vi "Example_OE1311&OE1351 Trig in.vi"() -> ()   [LabVIEW 2011]
panel:
  in  "Parameter Index":u16(ring) items=["X", "Y", "R", "θ", "XD1", "YD1", "RD1", "θD1", "XD2", "YD2", "RD2", "θD2", "XD3", "YD3", "RD3", "θD3", "XD4", "YD4", "RD4", "θD4", "XD5", "YD5", "RD5", "θD5", "XD6", "YD6", "RD6", "θD6", "XD7", "YD7", "RD7", "θD7", "X_Noise", "Y_Noise", "Frequency", "AUX-IN1", "AUX-IN2"]
  in  "Trig Mode":u8(ring) items=["Ext_Rissing_Edge", "Ext_Falling_Edge", "Ext_Bilateral_Edge", "Ext_High_Level", "Ext_Low_Level"]
  in  "Trig Source":u8(ring) items=["Internal", "Aux-in1", "Aux-in2"]
  out "Wave":dbl(graph)
  out "loss count":i32=-1
  out "Group":u32
  out "Error out":errorcluster caption="error out"
  in  "function":T1(ring)
  in  "Connect":bool
  in  "Port":u32=10001
  in  "Timeout":u32=100
  in  "IP Address":string="192.168.1.1"
  in  "选项卡控件":enum32{"选项卡 "}(tab)
  in  "Sweep Mode":u16(ring) items=["Linear", "Log"]
  in  "Start Frequency(Hz)":dbl=1000.0 min=1e-05 max=60000000.0 format="%#.3f"
  in  "Stop Frequency(Hz)":dbl=5000.0 min=1e-05 max=60000000.0 format="%#.3f"
  in  "Linear Step Frequency(Hz)":dbl=1000.0 min=1e-05 max=60000000.0 format="%#.3f"
  in  "Log Step Percent(%)":dbl=10.0 min=-100.0 max=100.0 format="%#.2f"
  in  "Step Time(ms)":i32=1000 min=50 max=100000
  in  "Sweep Run Mode":u16(ring) items=["Stop", "Singal", "Loop"]
  in  "Interval Count":u32=1 min=1 max=100000
  in  "Ref_Source":u8(ring) items=["External", "Internal"]
  in  "Sweep":u16(ring) items=["OFF", "ON"]
  out "data_buffer":dbl[][](array[numeric])
  out "cnt":u16
  # "Tel          :   +86-020-84133345\nWebsite  :   www.ssi-instrument.com\nE-mail     :   support@si-instrument.com"
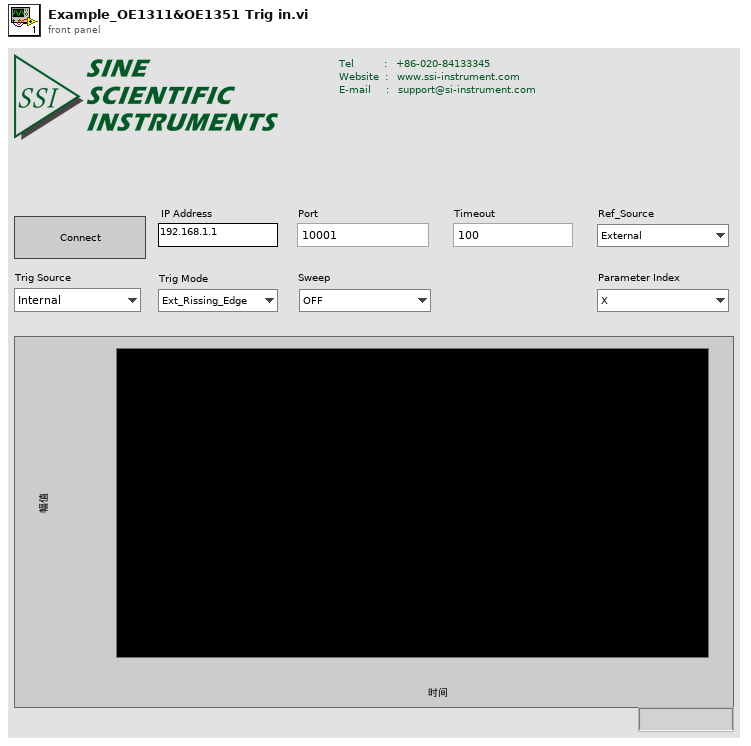
[diagram p1: front panel]
types:
  T1 = enum16{"initial", "Trig In Type", "Sample", "Ext_Sweep_Trig In", "Int_Sweep_Trig In"}
  T2 = enum8{"Enabled", "Disabled", "Disabled and Grayed Out"}
  T3 = cluster{"Port":u32, "Timeout":u32, "IP Address":string}
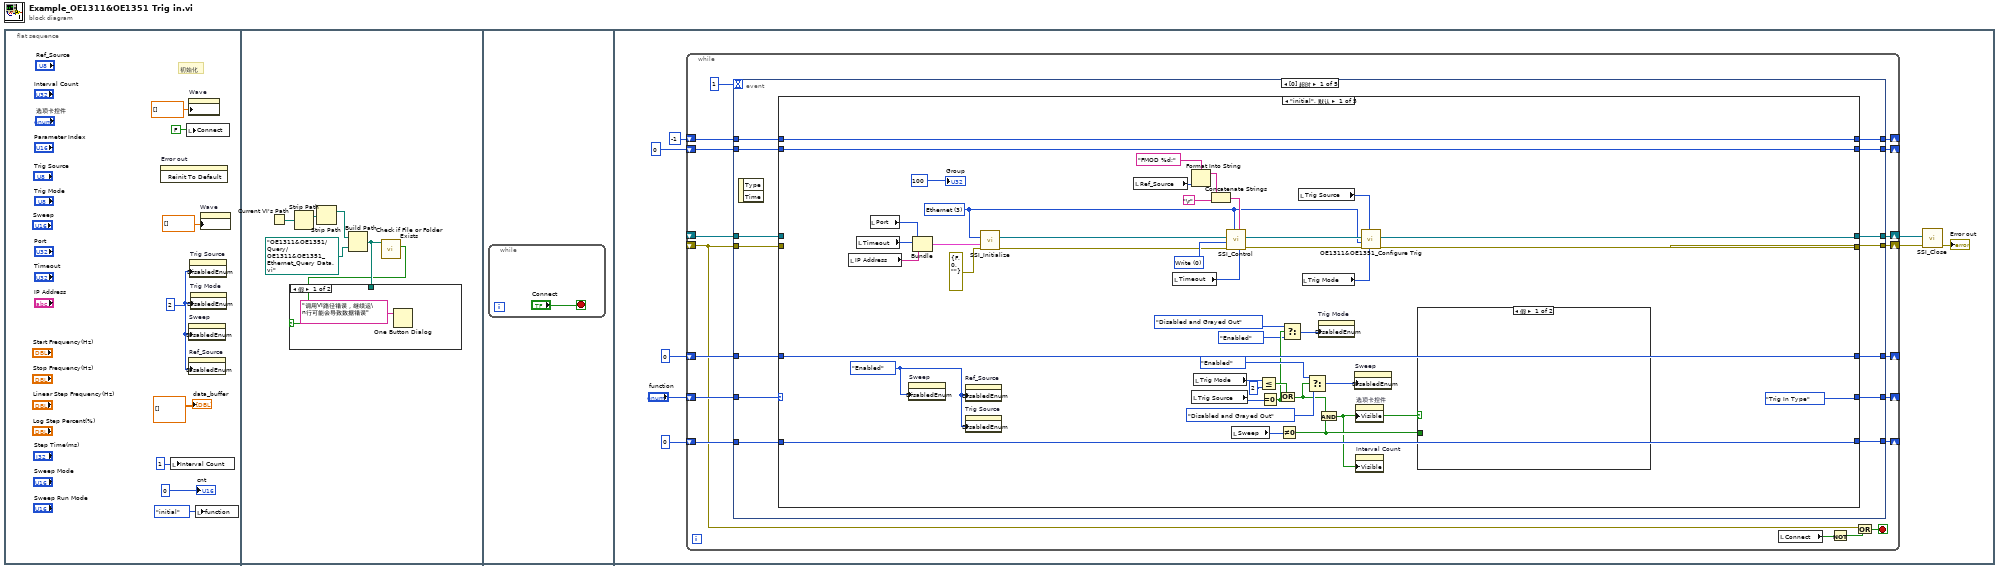
[diagram p0: block diagram]
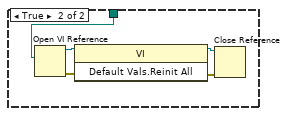
[diagram p2: hidden frame]
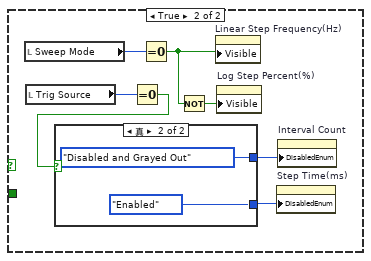
[diagram p3: hidden frame]
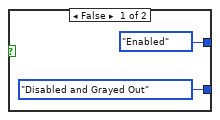
[diagram p4: hidden frame]
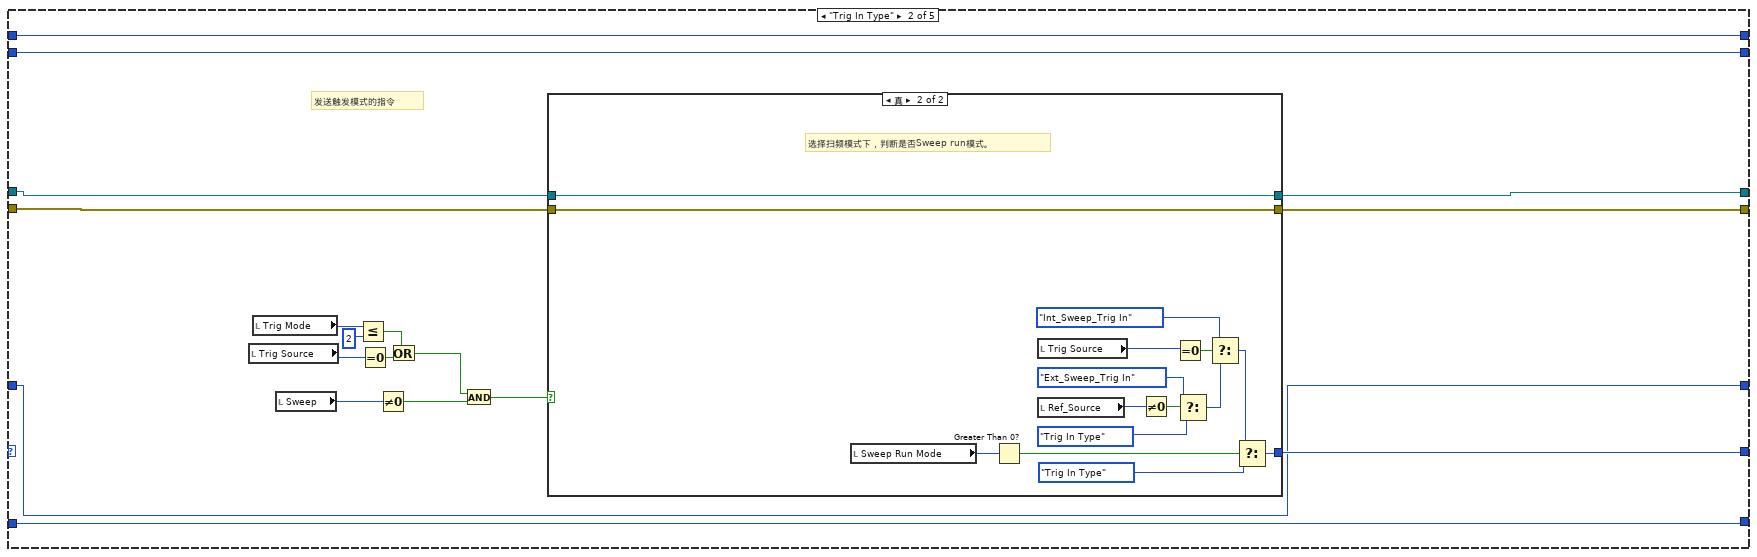
[diagram p5: hidden frame]
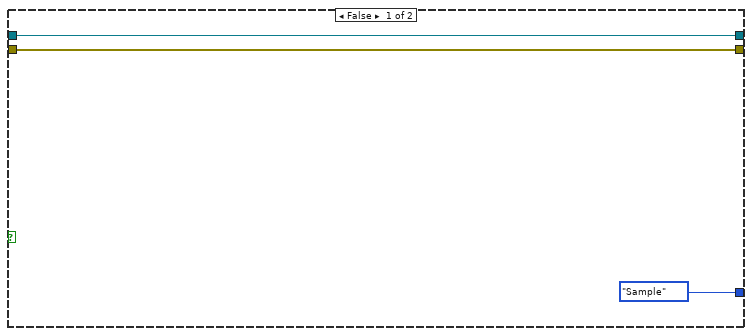
[diagram p6: hidden frame]
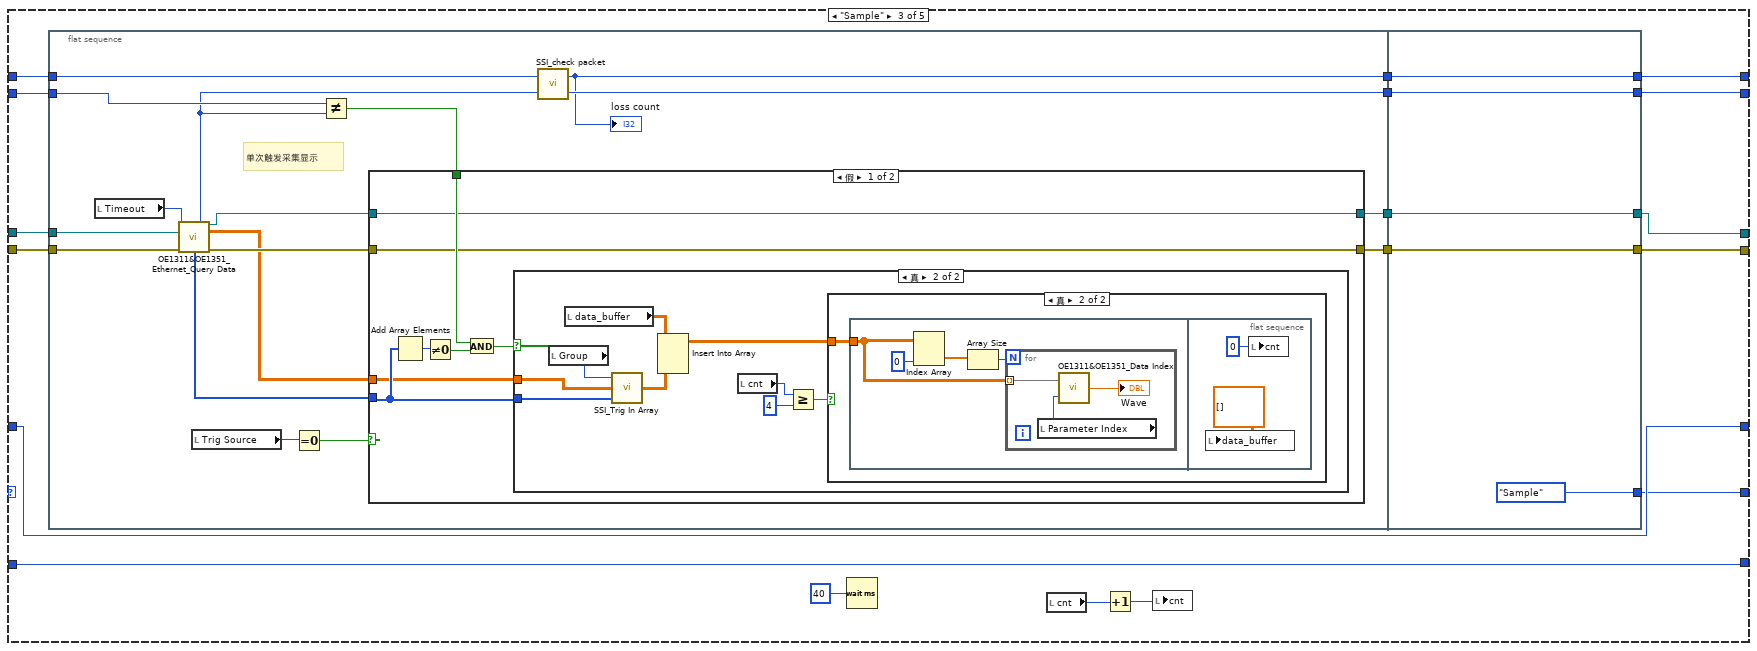
[diagram p7: hidden frame]
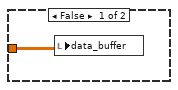
[diagram p9: hidden frame]
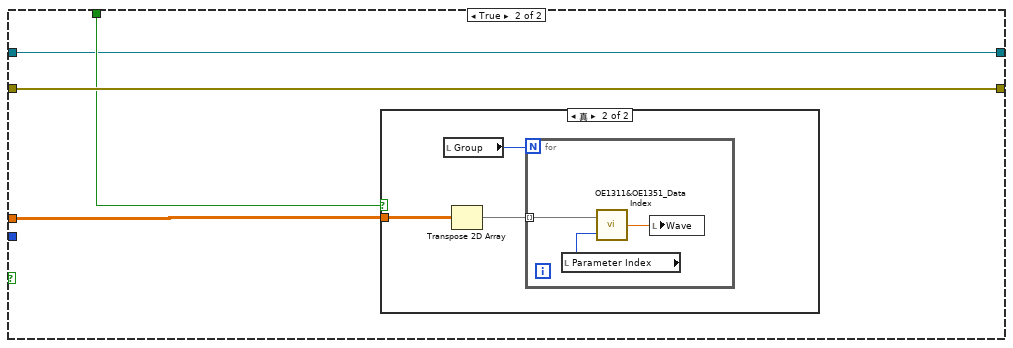
[diagram p10: hidden frame]
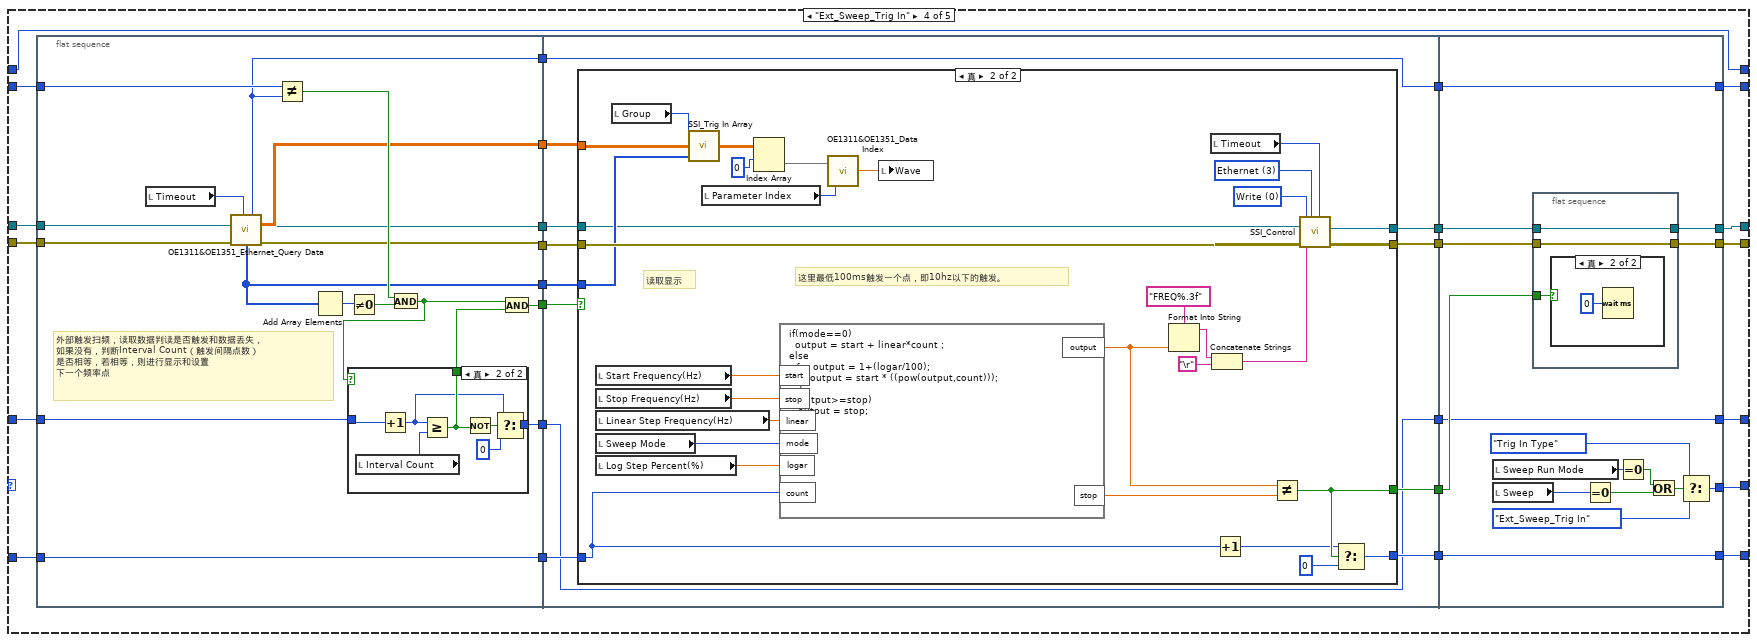
[diagram p12: hidden frame]
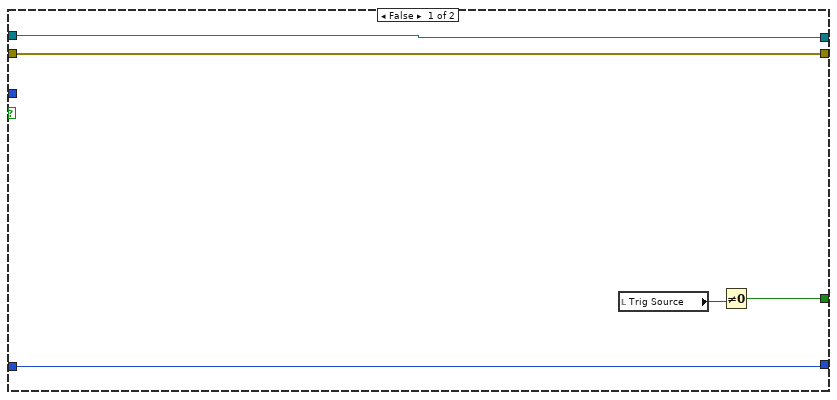
[diagram p14: hidden frame]
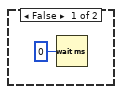
[diagram p15: hidden frame]
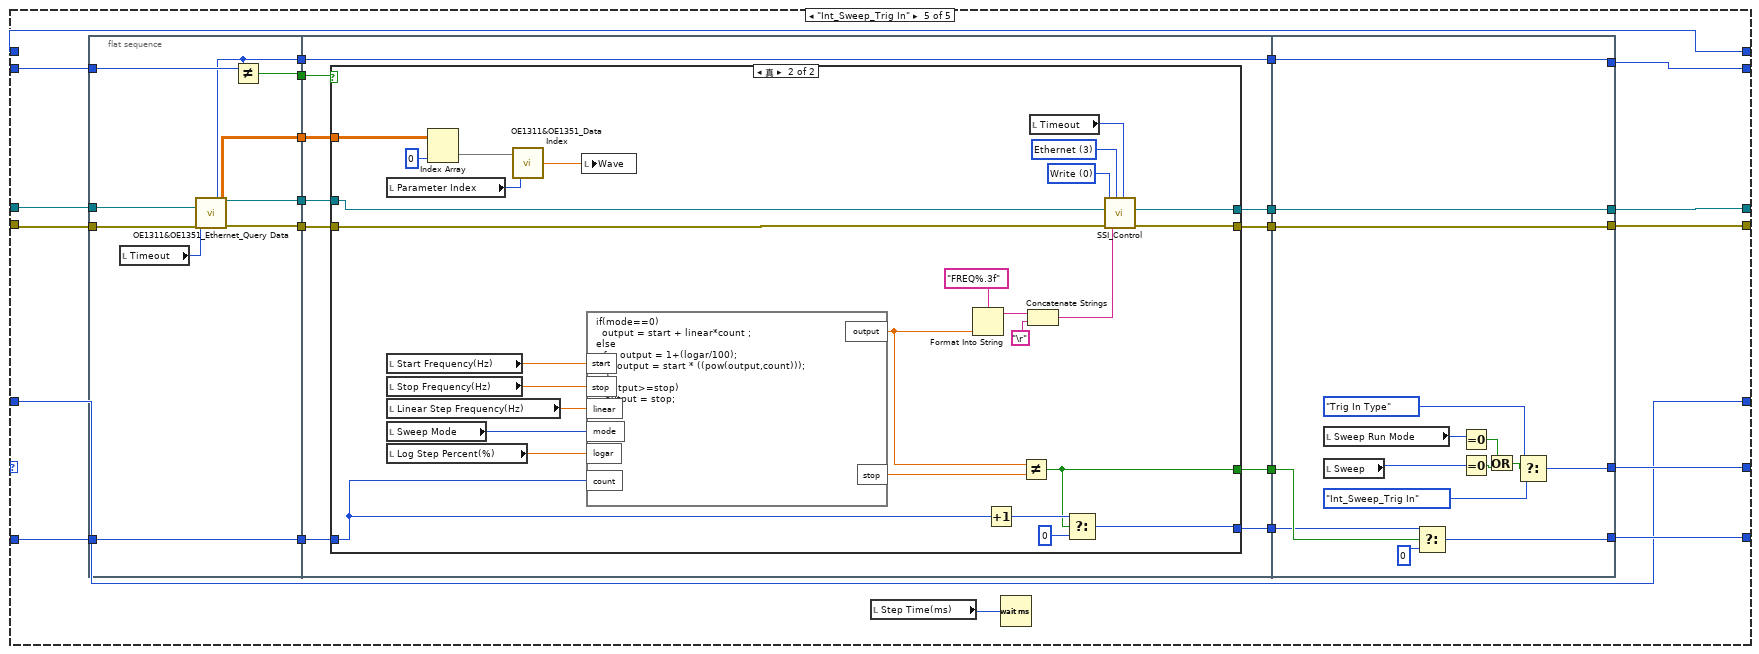
[diagram p16: hidden frame]
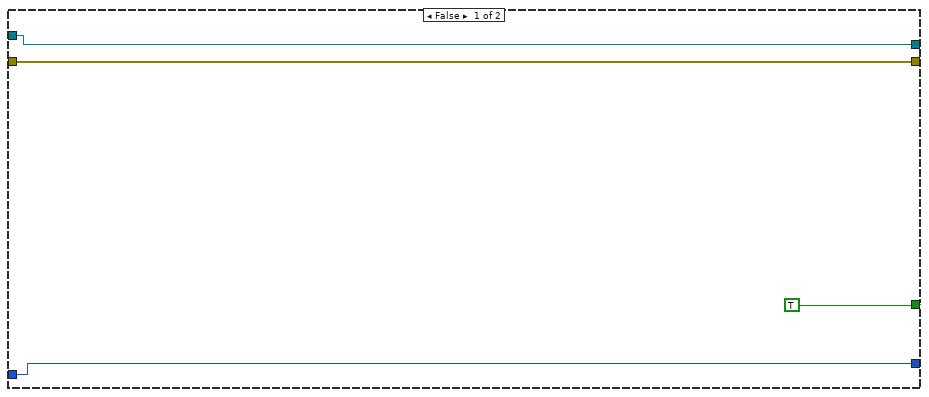
[diagram p17: hidden frame]
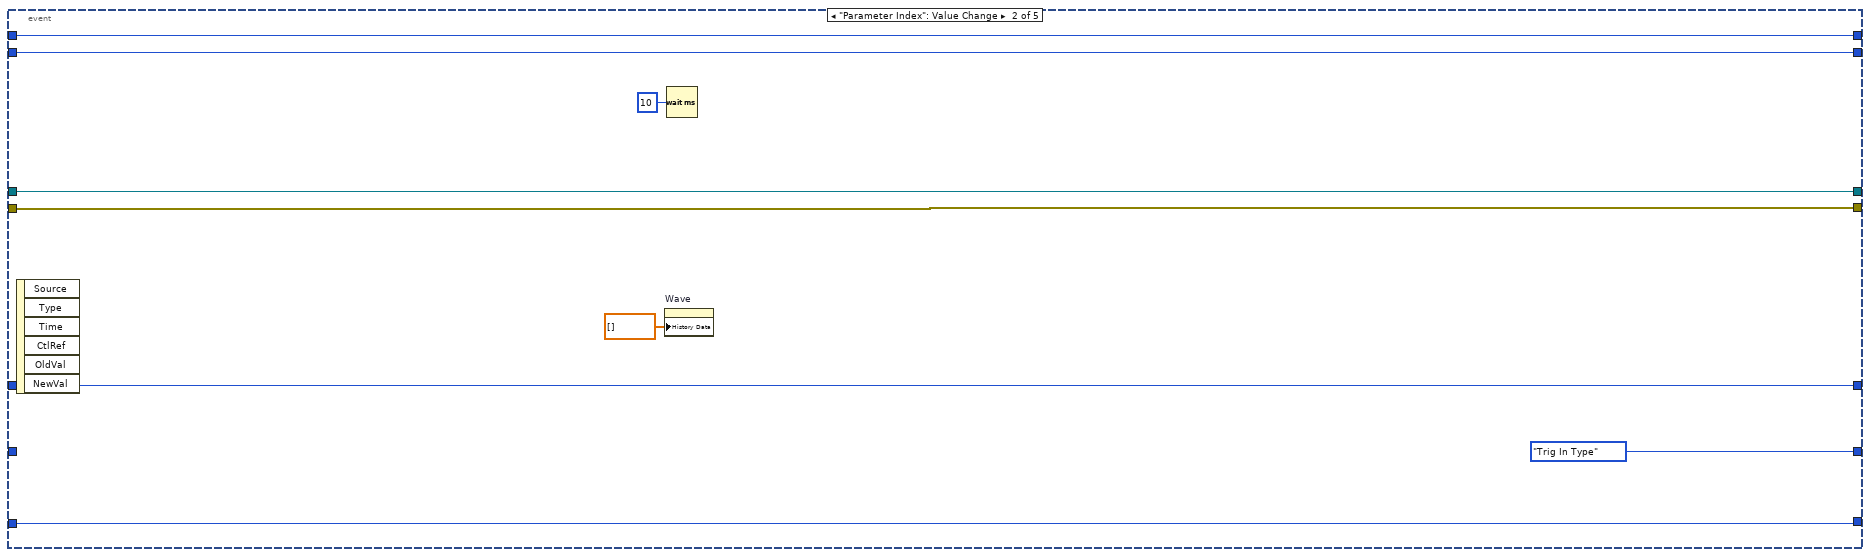
[diagram p18: hidden frame]
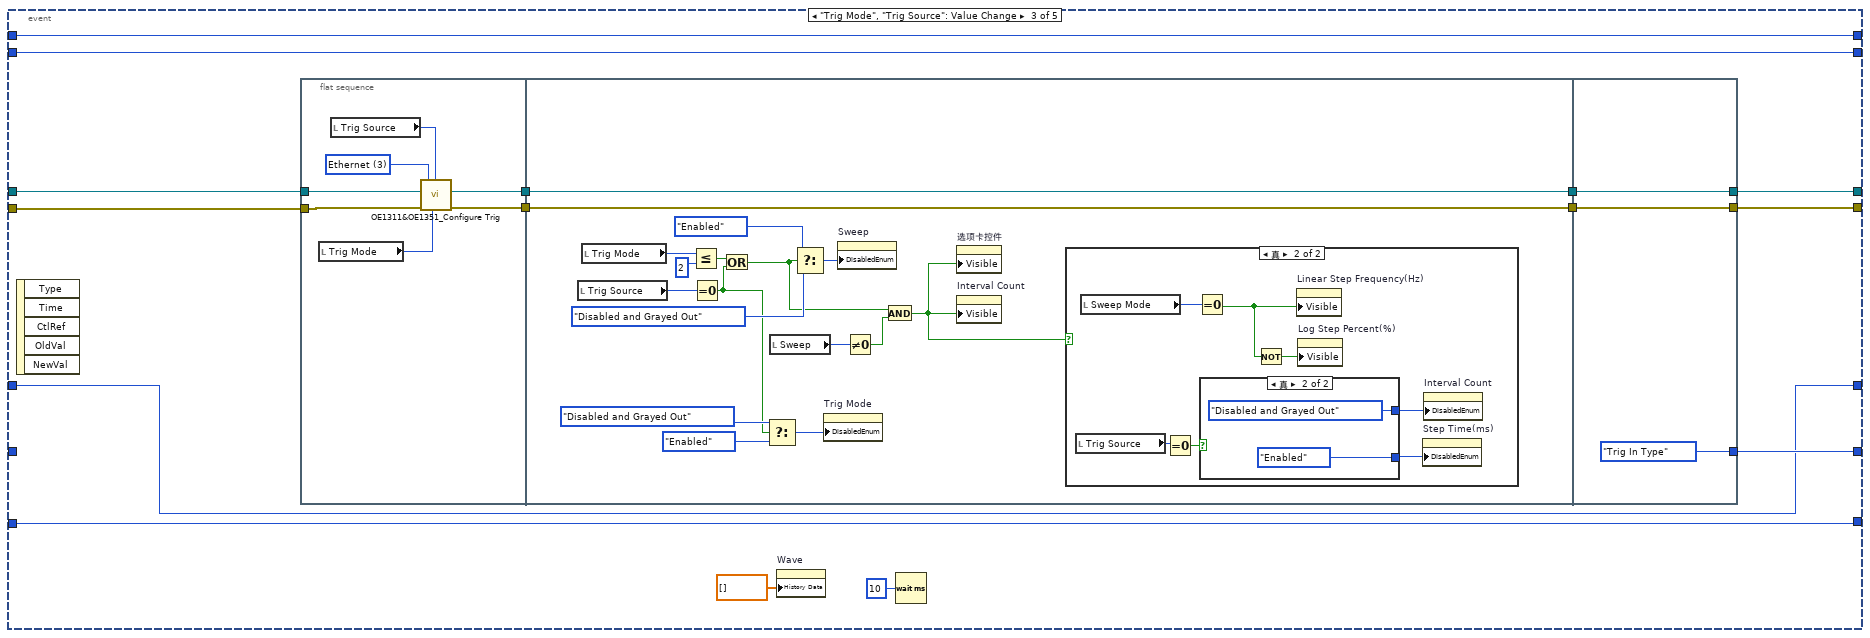
[diagram p19: hidden frame]
diagram:
  n1 = flat-sequence {
    frame #0 {
      w1 = 2
      # "初始化"
      n2 = invoke on="Error out" class="Clust (严格)" method="Reinit To Default"() -> ()  [unwired: 3 in, 3 out]
      n3 = local write "Interval Count"(u32 1 ("Interval Count")) -> ()
      n4 = local write "Connect"(FALSE ("Connect")) -> ()
      n5 = property on="Wave" class="WFChart (严格)"("History Data"=dbl[] [] ("历史数据")) -> ()  [unwired: 2 in, 2 out]
      n6 = property on="Sweep" class="Ring (严格)"("DisabledEnum"=w1) -> ()  [unwired: 2 in, 2 out]
      n7 = property on="Ref_Source" class="Ring (严格)"("DisabledEnum"=w1) -> ()  [unwired: 2 in, 2 out]
      n8 = property on="Trig Source" class="Ring (严格)"("DisabledEnum"=w1) -> ()  [unwired: 2 in, 2 out]
      n9 = property on="Trig Mode" class="Ring (严格)"("DisabledEnum"=w1) -> ()  [unwired: 2 in, 2 out]
      n10 = local write "function"(T1."initial" ("function")) -> ()
      n11 = property on="Wave" class="WFChart (严格)"("History Data"=dbl[] [] ("历史数据")) -> ()  [unwired: 2 in, 2 out]
      "data_buffer" <- dbl[][] []
      "cnt" <- 0
    }
    frame #1 {
      n12 = Current VI's Path() -> (path=w10:path)
      n13 = Strip Path(path=w10) -> (stripped path=w9:path)  [unwired: 1 out]
      n14 = Strip Path(path=w9) -> (stripped path=w11:path)  [unwired: 1 out]
      n15 = Build Path(base path=w11, name or relative path=path "OE1311&OE1351/Query/OE1311&OE1351_Ethernet_Query Data.vi") -> (appended path=w14:path)
      n16 = call <vilib>:"Check if File or Folder Exists.vi"("path"=w14) -> ("file or folder exists?"=w12:bool)  [unwired: 8 in, 2 out]
      n17 = case shown="假" w12 {
        tunnel: w14 -> [_ w20]
        frame False {
          n18 = One Button Dialog(message="调用VI路径错误，继续运\n行可能会导致数据错误" ("消息")) -> ()  [unwired: 1 in, 1 out]
        }
        frame True {
          n19 = Open VI Reference(vi path=w20) -> (vi reference=w17:refnum<vi>, error out=w16:errorcluster)  [unwired: 5 in]
          n20 = invoke class="VI" method="Default Vals.Reinit All"(reference=w17, error in=w16) -> (reference out=w19:refnum<vi>, error out=w18:errorcluster)  [unwired: 1 in, 1 out]
          n21 = Close Reference(reference=w19, error in (no error)=w18) -> ()  [unwired: 1 out]
        }
      }
    }
    frame #2 {
      n22 = while {
        stop <- "Connect" stop-if-true
      }
    }
    frame #3 {
      n23 = while {
        shift-right: [w43] -> _
        shift-left: "function" -> [w44]
        shift-right: [w41] -> _
        shift-left: 0 ("f") -> [w42]
        shift-right: [w38] -> _
        shift-left: 0 -> [w39]
        shift-right: [w35] -> _
        shift-left: 0 -> [w36]
        shift-right: [w45] -> w28
        shift-left: _ -> [w34]
        shift-right: [w33] -> w24
        shift-left: _ -> [w32]
        shift-right: [w30] -> _
        shift-left: -1 ("loss count") -> [w31]
        stop <- w46 stop-if-true
        n24 = event shown="[0] 超时" {
          selector: _ -> [_ _ _ _ _]
          dyn-events: _ -> [_ _ _ _ _]
          timeout: 1 -> [_ _ _ _ _]
          tunnel: [w61 w446 w452 w509 w526] -> w45
          tunnel: w34 -> [w60 w446 w456 w510 w526]
          tunnel: w44 -> [w59 _ _ w513 _]
          tunnel: [w58 T1."Trig In Type" ("function") w458 w513 T1."Trig In Type" ("function")] -> w43
          tunnel: w42 -> [w57 w448 w463 w514 w522]
          tunnel: [w56 w448 w463 w514 w522] -> w41
          tunnel: w39 -> [w55 w444 w462 w511 w524]
          tunnel: [w54 w444 w462 w511 w524] -> w38
          tunnel: w36 -> [w53 w443 w457 w512 w521]
          tunnel: [w52 w443 w457 w512 w521] -> w35
          tunnel: [w51 w441 w449 w507 w525] -> w33
          tunnel: w32 -> [w50 w441 w455 w508 w525]
          tunnel: w31 -> [w49 w440 w459 w503 w523]
          tunnel: [w48 w440 w459 w503 w523] -> w30
          event Timeout {
            n25 = event-data() -> ()  [unwired: 1 in, 2 out]
            n26 = case shown="\"initial\", 默认" w59 {
              tunnel: w60 -> [_ w133 w168 w254 w360]
              tunnel: [w93 w132 w161 w252 w370] -> w61
              tunnel: [T1."Trig In Type" ("function") w131 w166 w243 w368] -> w58
              tunnel: w57 -> [w103 w130 w169 w253 w369]
              tunnel: [w103 w130 w169 w251 w367] -> w56
              tunnel: w55 -> [w101 w129 w165 w250 w372]
              tunnel: [w101 w129 w163 w249 w371] -> w54
              tunnel: w53 -> [w102 w128 w167 w237 w366]
              tunnel: [w102 w128 w167 w234 w366] -> w52
              tunnel: [w94 w123 w154 w231 w352] -> w51
              tunnel: w50 -> [_ w124 w156 w233 w356]
              tunnel: w49 -> [w85 w122 w159 w230 w351]
              tunnel: [w85 w122 w153 w230 w351] -> w48
              frame "initial", Default {
                w64 = u16 3 items=["USB", "RS232", "GPIB", "Ethernet"] ("Remote Mode")
                w82 = T2."Enabled" ("禁用")
                w87 = u16 0 items=["Write", "Read"] ("Control")
                n27 = local read "IP Address"() -> (w90:string)
                n28 = local read "Timeout"() -> (w91:u32)
                n29 = local read "Port"() -> (w92:u32)
                n30 = property on="Sweep" class="Ring (严格)"("DisabledEnum"=w82) -> ()  [unwired: 2 in, 2 out]
                n31 = Bundle("Port"=w92, "Timeout"=w91, "IP Address"=w90) -> (w89:T3)  [unwired: 1 in]
                n32 = property on="Ref_Source" class="Ring (严格)"("DisabledEnum"=w82) -> ()  [unwired: 2 in, 2 out]
                n33 = property on="Trig Source" class="Ring (严格)"("DisabledEnum"=w82) -> ()  [unwired: 2 in, 2 out]
                n34 = call "SSI_Initialize.vi"("Remote Mode"=w64, "Ethernet"=w89, "error in (no error)"=errorcluster {"status"=FALSE, "code"=0, "source"=""}) -> ("connection ID(Ethernet)"=w63:refnum<k5>, "error out"=w62:errorcluster)  [unwired: 10 in, 1 out]
                n35 = local read "Ref_Source"() -> (w99:u8)
                n36 = local read "Timeout"() -> (w83:u32)
                n37 = Format Into String(format string="FMOD %d;" ("格式字符串"), w99) -> (resulting string=w100:string)  [unwired: 2 in, 1 out]
                n38 = local read "Trig Source"() -> (w72:u8)
                n39 = local read "Trig Mode"() -> (w70:u8)
                n40 = Concatenate Strings(w100, "\r") -> (w86:string)
                n41 = call "SSI_Control.vi"("Tineout"=w83, "Write Buffer"=w86, "Remote Mode"=w64, "Error in (no error)"=w62, "Control"=w87, "Connection ID in"=w63) -> ("Error out"=w95:errorcluster, "Connection ID out"=w96:refnum<k5>)  [unwired: 2 in, 2 out]
                n42 = local read "Sweep"() -> (w76:u16)
                n43 = Less Or Equal?(x=w70, y=u8 2) -> (x <= y?=w71:bool)
                n44 = Equal To 0?(x=w72) -> (x = 0?=w68:bool)
                n45 = Or(x=w71, y=w68) -> (x .or. y?=w69:bool)
                n46 = Not Equal To 0?(x=w76) -> (x != 0?=w79:bool)
                n47 = Select(t=T2."Disabled and Grayed Out" ("禁用"), s=w68, f=T2."Enabled" ("禁用")) -> (s? t:f=w67:T2)
                n48 = local read "Trig Source"() -> (w80:u8)
                n49 = local read "Trig Mode"() -> (w81:u8)
                n50 = Select(t=T2."Enabled" ("禁用"), s=w69, f=T2."Disabled and Grayed Out") -> (s? t:f=w74:T2)
                n51 = property on="Trig Mode" class="Ring (严格)"("DisabledEnum"=w67) -> ()  [unwired: 2 in, 2 out]
                n52 = And(x=w69, y=w79) -> (x .and. y?=w78:bool)
                n53 = property on="Sweep" class="Ring (严格)"("DisabledEnum"=w74) -> ()  [unwired: 2 in, 2 out]
                n54 = property on="选项卡控件" class="TabCtl (严格)"("Visible"=w78) -> ()  [unwired: 2 in, 2 out]
                n55 = property on="Interval Count" class="DigNum (严格)"("Visible"=w78) -> ()  [unwired: 2 in, 2 out]
                n56 = call "OE1311&OE1351_Configure Trig.vi"("Trig Mode"=w81, "Trig Source"=w80, "Error in (no error)"=w95, "Remote Mode"=w64, "Connection ID in"=w96) -> ("Error out"=w93:errorcluster, "Connection ID out"=w94:refnum<k5>)  [unwired: 3 in, 2 out]
                n57 = case shown="假" w78 {
                  tunnel: w79 -> [_ _]
                  frame False {
                  }
                  frame True {
                    n58 = local read "Sweep Mode"() -> (w110:u16)
                    n59 = local read "Trig Source"() -> (w105:u8)
                    n60 = Equal To 0?(x=w105) -> (x = 0?=w106:bool)
                    n61 = case shown="真" w106 {
                      tunnel: [T2."Disabled and Grayed Out" ("禁用") T2."Enabled" ("禁用")] -> w108
                      tunnel: [T2."Enabled" ("禁用") T2."Disabled and Grayed Out" ("禁用")] -> w107
                      frame False {
                      }
                      frame True {
                      }
                    }
                    n62 = Equal To 0?(x=w110) -> (x = 0?=w111:bool)
                    n63 = Not(x=w111) -> (.not. x?=w109:bool)
                    n64 = property on="Linear Step Frequency(Hz)" class="DigNum (严格)"("Visible"=w111) -> ()  [unwired: 2 in, 2 out]
                    n65 = property on="Log Step Percent(%)" class="DigNum (严格)"("Visible"=w109) -> ()  [unwired: 2 in, 2 out]
                    n66 = property on="Step Time(ms)" class="DigNum (严格)"("DisabledEnum"=w108) -> ()  [unwired: 2 in, 2 out]
                    n67 = property on="Interval Count" class="DigNum (严格)"("DisabledEnum"=w107) -> ()  [unwired: 2 in, 2 out]
                  }
                }
                "Group" <- 100
              }
              frame "Trig In Type" {
                # "发送触发模式的指令"
                n68 = local read "Trig Source"() -> (w118:u8)
                n69 = local read "Trig Mode"() -> (w121:u8)
                n70 = local read "Sweep"() -> (w126:u16)
                n71 = Less Or Equal?(x=w121, y=u8 2) -> (x <= y?=w119:bool)
                n72 = Equal To 0?(x=w118) -> (x = 0?=w120:bool)
                n73 = Not Equal To 0?(x=w126) -> (x != 0?=w125:bool)
                n74 = Or(x=w119, y=w120) -> (x .or. y?=w116:bool)
                n75 = And(x=w116, y=w125) -> (x .and. y?=w127:bool)
                n76 = case shown="真" w127 {
                  tunnel: [w136 w147] -> w132
                  tunnel: w133 -> [w136 w147]
                  tunnel: [T1."Sample" ("function") w150] -> w131
                  tunnel: w124 -> [w134 w138]
                  tunnel: [w134 w138] -> w123
                  frame False {
                  }
                  frame True {
                    # "选择扫频模式下，判断是否Sweep run模式。"
                    n77 = local read "Sweep Run Mode"() -> (w148:u16)
                    n78 = Greater Than 0?(x=w148) -> (x > 0?=w151:bool)
                    n79 = local read "Trig Source"() -> (w137:u8)
                    n80 = local read "Ref_Source"() -> (w146:u8)
                    n81 = Not Equal To 0?(x=w146) -> (x != 0?=w145:bool)
                    n82 = Equal To 0?(x=w137) -> (x = 0?=w143:bool)
                    n83 = Select(t=T1."Ext_Sweep_Trig In" ("function"), s=w145, f=T1."Trig In Type" ("function")) -> (s? t:f=w144:T1)
                    n84 = Select(t=T1."Int_Sweep_Trig In" ("function"), s=w143, f=w144) -> (s? t:f=w149:T1)
                    n85 = Select(t=w149, s=w151, f=T1."Trig In Type" ("function")) -> (s? t:f=w150:T1)
                  }
                }
              }
              frame "Sample" {
                n86 = flat-sequence {
                  tunnel: w168 -> [w185]
                  tunnel: w165 -> [w182]
                  tunnel: [w179] -> w164
                  tunnel: [w180] -> w162
                  tunnel: w159 -> [w178]
                  tunnel: w156 -> [w176]
                  tunnel: [w174] -> w155
                  tunnel: [w173] -> w152
                  tunnel: w164 -> [w228]
                  tunnel: w162 -> [w227]
                  tunnel: [T1."Sample" ("function")] -> w166
                  tunnel: [w228] -> w163
                  tunnel: [w227] -> w161
                  tunnel: w155 -> [w225]
                  tunnel: [w225] -> w154
                  tunnel: [w224] -> w153
                  tunnel: w152 -> [w224]
                  frame #0 {
                    # "单次触发采集显示"
                    n87 = local read "Timeout"() -> (w172:u32)
                    n88 = call "OE1311&OE1351_Ethernet_Query Data.vi"("Connection ID in"=w176, "Timeout"=w172, "Error in (no error)"=w185) -> ("Buffer Count"=w179:u8, "Connection ID out"=w175:refnum<k5>, "Total Date Array"=w177:dbl[][], "Trig_Count"=w183:u8[], "Error out"=w181:errorcluster)  [unwired: 5 in, 3 out]
                    n89 = local read "Trig Source"() -> (w171:u8)
                    n90 = Equal To 0?(x=w171) -> (x = 0?=w184:bool)
                    n91 = Not Equal?(x=w182, y=w179) -> (x != y?=w170:bool)
                    n92 = case shown="假" w184 {
                      tunnel: w177 -> [w189 w216]
                      tunnel: w183 -> [w192 _]
                      tunnel: w170 -> [w188 w215]
                      tunnel: w181 -> [w186 w217]
                      tunnel: [w186 w217] -> w180
                      tunnel: w175 -> [w187 w214]
                      tunnel: [w187 w214] -> w174
                      frame False {
                        n93 = Add Array Elements(numeric array=w192) -> (sum=w193:u8)
                        n94 = Not Equal To 0?(x=w193) -> (x != 0?=w191:bool)
                        n95 = And(x=w188, y=w191) -> (x .and. y?=w190:bool)
                        n96 = case shown="真" w190 {
                          tunnel: w189 -> [_ w202]
                          tunnel: w192 -> [_ w201]
                          frame False {
                          }
                          frame True {
                            n97 = local read "Group"() -> (w200:u32)
                            n98 = local read "data_buffer"() -> (w199:dbl[][])
                            n99 = call "SSI_Trig In Array.vi"("Trig_Count"=w201, "Input Array"=w202, "Group"=w200) -> ("Output Array"=w198:dbl[][])
                            n100 = Insert Into Array(array=w199, new element=w198) -> (w197:dbl[][])  [unwired: 2 in]
                            n101 = local read "cnt"() -> (w196:u16)
                            n102 = Greater Or Equal?(x=w196, y=u16 4) -> (x >= y?=w194:bool)
                            n103 = case shown="真" w194 {
                              tunnel: w197 -> [w203 w204]
                              frame False {
                                n104 = local write "data_buffer"(w203) -> ()
                              }
                              frame True {
                                n105 = flat-sequence {
                                tunnel: w204 -> [w206]
                                frame #0 {
                                n106 = Index Array(array=w206, index (col)=0 ("禁用的索引 (列)")) -> (element=w205:dbl[])  [unwired: 1 in]
                                n107 = Array Size(array=w205) -> (size(s)=w208:i32)
                                n108 = for {
                                N: w208 -> [_]
                                tunnel: w206 -> [w210] mode=indexing
                                n109 = local read "Parameter Index"() -> (w209:u16)
                                n110 = call "OE1311&OE1351_Data Index.vi"("Parameter Type"=w209, "Input Date Array"=w210) -> ("Parameter"=→"Wave":dbl)
                                }
                                }
                                frame #1 {
                                n111 = local write "data_buffer"(dbl[][] [] ("data_buffer")) -> ()
                                n112 = local write "cnt"(u16 0 ("cnt")) -> ()
                                }
                                }
                              }
                            }
                          }
                        }
                      }
                      frame True {
                        n113 = case shown="真" w215 {
                          tunnel: w216 -> [_ w220]
                          frame False {
                          }
                          frame True {
                            n114 = local read "Group"() -> (w219:u32)
                            n115 = Transpose 2D Array(2D array=w220) -> (transposed array=w218:dbl[][])
                            n116 = for {
                              N: w219 -> [_]
                              tunnel: w218 -> [w223] mode=indexing
                              n117 = local read "Parameter Index"() -> (w221:u16)
                              n118 = call "OE1311&OE1351_Data Index.vi"("Parameter Type"=w221, "Input Date Array"=w223) -> ("Parameter"=w222:dbl)
                              n119 = local write "Wave"(w222) -> ()
                            }
                          }
                        }
                      }
                    }
                    n120 = call "SSI_check packet.vi"("input"=w179, "input loss"=w178) -> ("loss count"=w173:i32)  [unwired: 1 out]
                    "loss count" <- w173
                  }
                  frame #1 {
                  }
                }
                n121 = Wait (ms)(milliseconds to wait=40) -> ()  [unwired: 1 out]
                n122 = local read "cnt"() -> (w157:u16)
                n123 = Increment(x=w157) -> (x+1=w158:u16)
                n124 = local write "cnt"(w158) -> ()
              }
              frame "Ext_Sweep_Trig In" {
                n125 = flat-sequence {
                  tunnel: w254 -> [w271]
                  tunnel: w253 -> [w269]
                  tunnel: w250 -> [w272]
                  tunnel: [w269] -> w248
                  tunnel: [w270] -> w247
                  tunnel: [w265] -> w241
                  tunnel: [w264] -> w240
                  tunnel: [w263] -> w239
                  tunnel: [w262] -> w238
                  tunnel: w237 -> [w260]
                  tunnel: [w258] -> w236
                  tunnel: w233 -> [w257]
                  tunnel: [w256] -> w229
                  tunnel: w247 -> [w283]
                  tunnel: w248 -> [w290]
                  tunnel: [w291] -> w246
                  tunnel: [w289] -> w245
                  tunnel: [w283] -> w244
                  tunnel: [w288] -> w242
                  tunnel: w241 -> [w292]
                  tunnel: w240 -> [w287]
                  tunnel: w239 -> [w286]
                  tunnel: w238 -> [w285]
                  tunnel: w236 -> [w284]
                  tunnel: [w284] -> w235
                  tunnel: [w282] -> w232
                  tunnel: w229 -> [w281]
                  tunnel: [w343] -> w249
                  tunnel: [w344] -> w251
                  tunnel: [w341] -> w252
                  tunnel: w246 -> [w342]
                  tunnel: w245 -> [w344]
                  tunnel: w244 -> [w343]
                  tunnel: [w338] -> w243
                  tunnel: w242 -> [w340]
                  tunnel: w235 -> [w339]
                  tunnel: [w339] -> w234
                  tunnel: w232 -> [w334]
                  tunnel: [w333] -> w231
                  frame #0 {
                    # "外部触发扫频，读取数据判读是否触发和数据丢失，\n如果没有，判断Interval Count（触发间隔点数）\n是否相等，若相等，则进行显示和设置\n下一个频率点"
                    n126 = local read "Timeout"() -> (w255:u32)
                    n127 = call "OE1311&OE1351_Ethernet_Query Data.vi"("Connection ID in"=w257, "Timeout"=w255, "Error in (no error)"=w271) -> ("Buffer Count"=w270:u8, "Connection ID out"=w256:refnum<k5>, "Total Date Array"=w264:dbl[][], "Trig_Count"=w263:u8[], "Error out"=w265:errorcluster)  [unwired: 5 in, 3 out]
                    n128 = Not Equal?(x=w272, y=w270) -> (x != y?=w267:bool)
                    n129 = Add Array Elements(numeric array=w263) -> (sum=w268:u8)
                    n130 = Not Equal To 0?(x=w268) -> (x != 0?=w266:bool)
                    n131 = And(x=w267, y=w266) -> (x .and. y?=w261:bool)
                    n132 = case shown="真" w261 {
                      tunnel: w260 -> [w273 w280]
                      tunnel: [_ w277] -> w259
                      tunnel: [w273 w274] -> w258
                      frame False {
                      }
                      frame True {
                        n133 = local read "Interval Count"() -> (w279:u32)
                        n134 = Increment(x=w280) -> (x+1=w276:i32)
                        n135 = Greater Or Equal?(x=w276, y=w279) -> (x >= y?=w277:bool)
                        n136 = Not(x=w277) -> (.not. x?=w278:bool)
                        n137 = Select(t=w276, s=w278, f=0) -> (s? t:f=w274:i32)
                      }
                    }
                    n138 = And(x=w261, y=w259) -> (x .and. y?=w262:bool)
                  }
                  frame #1 {
                    n139 = case shown="真" w285 {
                      tunnel: w292 -> [w297 w311]
                      tunnel: [w297 w313] -> w291
                      tunnel: w290 -> [w296 w319]
                      tunnel: [w296 w318] -> w289
                      tunnel: [w295 w317] -> w288
                      tunnel: w287 -> [_ w310]
                      tunnel: w286 -> [_ w308]
                      tunnel: w281 -> [w294 w305]
                      tunnel: [w294 w304] -> w282
                      frame False {
                        n140 = local read "Trig Source"() -> (w293:u8)
                        n141 = Not Equal To 0?(x=w293) -> (x != 0?=w295:bool)
                      }
                      frame True {
                        w301 = u16 3 items=["USB", "RS232", "GPIB", "Ethernet"] ("Remote Mode")
                        w303 = u16 0 items=["Write", "Read"] ("Control")
                        # "这里最低100ms触发一个点，即10hz以下的触发。"
                        # "读取显示"
                        n142 = local read "Start Frequency(Hz)"() -> (w325:dbl)
                        n143 = local read "Stop Frequency(Hz)"() -> (w324:dbl)
                        n144 = local read "Linear Step Frequency(Hz)"() -> (w323:dbl)
                        n145 = local read "Sweep Mode"() -> (w322:u16)
                        n146 = local read "Log Step Percent(%)"() -> (w321:dbl)
                        n147 = local read "Group"() -> (w309:u32)
                        n148 = call "SSI_Trig In Array.vi"("Trig_Count"=w308, "Input Array"=w310, "Group"=w309) -> ("Output Array"=w307:dbl[][])
                        n149 = local read "Parameter Index"() -> (w300:u16)
                        n150 = Index Array(array=w307, index (row)=0 ("索引 (行)")) -> (element=w306:dbl[])  [unwired: 1 in]
                        n151 = formula code="if(mode==0)\n  output = start + linear*count ;\nelse \n  {    output = 1+(logar/100);\n       output = start * ((pow(output,count)));\n   }\nif(output>=stop)\n   output = stop;"("start"=w325, "stop"=w324, "linear"=w323, "logar"=w321, "mode"=w322, "count"=w319) -> ("stop"=w320:dbl, "output"=w314:dbl)
                        n152 = call "OE1311&OE1351_Data Index.vi"("Parameter Type"=w300, "Input Date Array"=w306) -> ("Parameter"=w299:dbl)
                        n153 = local write "Wave"(w299) -> ()
                        n154 = Format Into String(format string="FREQ%.3f" ("格式字符串"), w314) -> (resulting string=w327:string)  [unwired: 2 in, 1 out]
                        n155 = local read "Timeout"() -> (w302:u32)
                        n156 = Concatenate Strings(w327, "\r") -> (w312:string)
                        n157 = Increment(x=w319) -> (x+1=w316:i32)
                        n158 = Not Equal?(x=w314, y=w320) -> (x != y?=w317:bool)
                        n159 = call "SSI_Control.vi"("Tineout"=w302, "Write Buffer"=w312, "Remote Mode"=w301, "Error in (no error)"=w311, "Control"=w303, "Connection ID in"=w305) -> ("Error out"=w313:errorcluster, "Connection ID out"=w304:refnum<k5>)  [unwired: 2 in, 2 out]
                        n160 = Select(t=w316, s=w317, f=0) -> (s? t:f=w318:i32)
                      }
                    }
                  }
                  frame #2 {
                    n161 = local read "Sweep Run Mode"() -> (w329:u16)
                    n162 = local read "Sweep"() -> (w337:u16)
                    n163 = flat-sequence {
                      tunnel: [w347] -> w341
                      tunnel: w342 -> [w347]
                      tunnel: w340 -> [w346]
                      tunnel: [w345] -> w333
                      tunnel: w334 -> [w345]
                      frame #0 {
                        n164 = case shown="真" w346 {
                          frame False {
                            n165 = Wait (ms)(milliseconds to wait=u32 0 ("等待时间（毫秒）")) -> ()  [unwired: 1 out]
                          }
                          frame True {
                            n166 = Wait (ms)(milliseconds to wait=u32 0 ("等待时间（毫秒）")) -> ()  [unwired: 1 out]
                          }
                        }
                      }
                    }
                    n167 = Equal To 0?(x=w337) -> (x = 0?=w331:bool)
                    n168 = Equal To 0?(x=w329) -> (x = 0?=w330:bool)
                    n169 = Or(x=w330, y=w331) -> (x .or. y?=w332:bool)
                    n170 = Select(t=T1."Trig In Type" ("function"), s=w332, f=T1."Ext_Sweep_Trig In" ("function")) -> (s? t:f=w338:T1)
                  }
                }
              }
              frame "Int_Sweep_Trig In" {
                n171 = flat-sequence {
                  tunnel: [w379] -> w365
                  tunnel: [w378] -> w363
                  tunnel: w372 -> [w382]
                  tunnel: w369 -> [w380]
                  tunnel: w360 -> [w377]
                  tunnel: [w381] -> w359
                  tunnel: [w380] -> w358
                  tunnel: w356 -> [w376]
                  tunnel: [w375] -> w355
                  tunnel: [w374] -> w354
                  tunnel: w365 -> [w392]
                  tunnel: [w392] -> w364
                  tunnel: w363 -> [w391]
                  tunnel: [w390] -> w362
                  tunnel: [w386] -> w361
                  tunnel: w359 -> [w389]
                  tunnel: w358 -> [w388]
                  tunnel: [w387] -> w357
                  tunnel: w355 -> [w385]
                  tunnel: w354 -> [w384]
                  tunnel: [w383] -> w353
                  tunnel: [w439] -> w371
                  tunnel: w364 -> [w439]
                  tunnel: [w438] -> w370
                  tunnel: w362 -> [w438]
                  tunnel: [w432] -> w368
                  tunnel: [w437] -> w367
                  tunnel: w361 -> [w435]
                  tunnel: w357 -> [w434]
                  tunnel: w353 -> [w429]
                  tunnel: [w429] -> w352
                  frame #0 {
                    n172 = local read "Timeout"() -> (w373:u32)
                    n173 = call "OE1311&OE1351_Ethernet_Query Data.vi"("Connection ID in"=w376, "Timeout"=w373, "Error in (no error)"=w377) -> ("Buffer Count"=w379:u8, "Connection ID out"=w374:refnum<k5>, "Total Date Array"=w375:dbl[][], "Error out"=w378:errorcluster)  [unwired: 5 in, 4 out]
                    n174 = Not Equal?(x=w382, y=w379) -> (x != y?=w381:bool)
                  }
                  frame #1 {
                    n175 = case shown="真" w389 {
                      tunnel: [w396 w406] -> w390
                      tunnel: w391 -> [w396 w407]
                      tunnel: w388 -> [w395 w418]
                      tunnel: [w395 w412] -> w387
                      tunnel: [TRUE w413] -> w386
                      tunnel: w385 -> [_ w404]
                      tunnel: w384 -> [w393 w403]
                      tunnel: [w393 w401] -> w383
                      frame False {
                      }
                      frame True {
                        w399 = u16 3 items=["USB", "RS232", "GPIB", "Ethernet"] ("Remote Mode")
                        w402 = u16 0 items=["Write", "Read"] ("Control")
                        n176 = local read "Parameter Index"() -> (w398:u16)
                        n177 = local read "Start Frequency(Hz)"() -> (w424:dbl)
                        n178 = local read "Stop Frequency(Hz)"() -> (w423:dbl)
                        n179 = local read "Linear Step Frequency(Hz)"() -> (w422:dbl)
                        n180 = local read "Sweep Mode"() -> (w421:u16)
                        n181 = local read "Log Step Percent(%)"() -> (w420:dbl)
                        n182 = Index Array(array=w404, index (col)=0 ("禁用的索引 (列)")) -> (element=w408:dbl[])  [unwired: 1 in]
                        n183 = call "OE1311&OE1351_Data Index.vi"("Parameter Type"=w398, "Input Date Array"=w408) -> ("Parameter"=w397:dbl)
                        n184 = local write "Wave"(w397) -> ()
                        n185 = formula code="if(mode==0)\n  output = start + linear*count ;\nelse \n  {    output = 1+(logar/100);\n       output = start * ((pow(output,count)));\n   }\nif(output>=stop)\n   output = stop;"("start"=w424, "stop"=w423, "linear"=w422, "logar"=w420, "mode"=w421, "count"=w418) -> ("stop"=w414:dbl, "output"=w410:dbl)
                        n186 = Format Into String(format string="FREQ%.3f" ("格式字符串"), w410) -> (resulting string=w415:string)  [unwired: 2 in, 1 out]
                        n187 = Increment(x=w418) -> (x+1=w419:i32)
                        n188 = Not Equal?(x=w410, y=w414) -> (x != y?=w413:bool)
                        n189 = Concatenate Strings(w415, "\r") -> (w405:string)
                        n190 = local read "Timeout"() -> (w400:u32)
                        n191 = Select(t=w419, s=w413, f=0) -> (s? t:f=w412:i32)
                        n192 = call "SSI_Control.vi"("Tineout"=w400, "Write Buffer"=w405, "Remote Mode"=w399, "Error in (no error)"=w407, "Control"=w402, "Connection ID in"=w403) -> ("Error out"=w406:errorcluster, "Connection ID out"=w401:refnum<k5>)  [unwired: 2 in, 2 out]
                      }
                    }
                  }
                  frame #2 {
                    n193 = local read "Sweep Run Mode"() -> (w425:u16)
                    n194 = local read "Sweep"() -> (w433:u16)
                    n195 = Select(t=w434, s=w435, f=u16 0) -> (s? t:f=w437:i32)
                    n196 = Equal To 0?(x=w425) -> (x = 0?=w426:bool)
                    n197 = Equal To 0?(x=w433) -> (x = 0?=w427:bool)
                    n198 = Or(x=w426, y=w427) -> (x .or. y?=w428:bool)
                    n199 = Select(t=T1."Trig In Type" ("function"), s=w428, f=T1."Int_Sweep_Trig In" ("function")) -> (s? t:f=w432:T1)
                  }
                }
                n200 = local read "Step Time(ms)"() -> (w350:i32)
                n201 = Wait (ms)(milliseconds to wait=w350) -> ()  [unwired: 1 out]
              }
            }
          }
          event "Parameter Index": Value Change {
            n202 = event-data() -> ()  [unwired: 1 in, 6 out]
            n203 = property on="Wave" class="WFChart (严格)"("History Data"=dbl[] [] ("历史数据")) -> ()  [unwired: 2 in, 2 out]
            n204 = Wait (ms)(milliseconds to wait=u32 10 ("等待时间（毫秒）")) -> ()  [unwired: 1 out]
          }
          event "Trig Mode", "Trig Source": Value Change {
            n205 = event-data() -> ()  [unwired: 1 in, 5 out]
            n206 = flat-sequence {
              tunnel: w456 -> [w469]
              tunnel: w455 -> [w470]
              tunnel: [w467] -> w453
              tunnel: [w466] -> w450
              tunnel: [w480] -> w454
              tunnel: w453 -> [w480]
              tunnel: [w479] -> w451
              tunnel: w450 -> [w479]
              tunnel: [T1."Trig In Type" ("function")] -> w458
              tunnel: w454 -> [w500]
              tunnel: [w500] -> w452
              tunnel: w451 -> [w499]
              tunnel: [w499] -> w449
              frame #0 {
                w468 = u16 3 items=["USB"=0, "Ethernet"=3] ("Remote Mode")
                n207 = local read "Trig Mode"() -> (w465:u8)
                n208 = local read "Trig Source"() -> (w464:u8)
                n209 = call "OE1311&OE1351_Configure Trig.vi"("Trig Mode"=w465, "Trig Source"=w464, "Error in (no error)"=w469, "Remote Mode"=w468, "Connection ID in"=w470) -> ("Error out"=w467:errorcluster, "Connection ID out"=w466:refnum<k5>)  [unwired: 3 in, 2 out]
              }
              frame #1 {
                n210 = local read "Trig Source"() -> (w476:u8)
                n211 = local read "Trig Mode"() -> (w475:u8)
                n212 = Less Or Equal?(x=w475, y=u8 2) -> (x <= y?=w478:bool)
                n213 = Equal To 0?(x=w476) -> (x = 0?=w471:bool)
                n214 = Or(x=w478, y=w471) -> (x .or. y?=w477:bool)
                n215 = Select(t=T2."Disabled and Grayed Out" ("禁用"), s=w471, f=T2."Enabled" ("禁用")) -> (s? t:f=w474:T2)
                n216 = local read "Sweep"() -> (w482:u16)
                n217 = Select(t=T2."Enabled" ("禁用"), s=w477, f=T2."Disabled and Grayed Out") -> (s? t:f=w486:T2)
                n218 = property on="Trig Mode" class="Ring (严格)"("DisabledEnum"=w474) -> ()  [unwired: 2 in, 2 out]
                n219 = property on="Sweep" class="Ring (严格)"("DisabledEnum"=w486) -> ()  [unwired: 2 in, 2 out]
                n220 = Not Equal To 0?(x=w482) -> (x != 0?=w481:bool)
                n221 = And(x=w477, y=w481) -> (x .and. y?=w483:bool)
                n222 = property on="选项卡控件" class="TabCtl (严格)"("Visible"=w483) -> ()  [unwired: 2 in, 2 out]
                n223 = property on="Interval Count" class="DigNum (严格)"("Visible"=w483) -> ()  [unwired: 2 in, 2 out]
                n224 = case shown="真" w483 {
                  frame False {
                  }
                  frame True {
                    n225 = local read "Trig Source"() -> (w488:u8)
                    n226 = local read "Sweep Mode"() -> (w493:u16)
                    n227 = Equal To 0?(x=w488) -> (x = 0?=w489:bool)
                    n228 = Equal To 0?(x=w493) -> (x = 0?=w494:bool)
                    n229 = case shown="真" w489 {
                      tunnel: [T2."Disabled and Grayed Out" ("禁用") T2."Enabled" ("禁用")] -> w491
                      tunnel: [T2."Enabled" ("禁用") T2."Disabled and Grayed Out" ("禁用")] -> w490
                      frame False {
                      }
                      frame True {
                      }
                    }
                    n230 = Not(x=w494) -> (.not. x?=w492:bool)
                    n231 = property on="Linear Step Frequency(Hz)" class="DigNum (严格)"("Visible"=w494) -> ()  [unwired: 2 in, 2 out]
                    n232 = property on="Log Step Percent(%)" class="DigNum (严格)"("Visible"=w492) -> ()  [unwired: 2 in, 2 out]
                    n233 = property on="Step Time(ms)" class="DigNum (严格)"("DisabledEnum"=w491) -> ()  [unwired: 2 in, 2 out]
                    n234 = property on="Interval Count" class="DigNum (严格)"("DisabledEnum"=w490) -> ()  [unwired: 2 in, 2 out]
                  }
                }
              }
              frame #2 {
              }
            }
            n235 = property on="Wave" class="WFChart (严格)"("History Data"=dbl[] [] ("历史数据")) -> ()  [unwired: 2 in, 2 out]
            n236 = Wait (ms)(milliseconds to wait=u32 10 ("等待时间（毫秒）")) -> ()  [unwired: 1 out]
          }
          event "Ref_Source": Value Change {
            w502 = u16 3 items=["USB", "RS232", "GPIB", "Ethernet"] ("Remote Mode")
            w518 = u16 0 items=["Write", "Read"] ("Control")
            n237 = event-data() -> ()  [unwired: 1 in, 5 out]
            n238 = local read "Ref_Source"() -> (w516:u8)
            n239 = Format Into String(format string="FMOD %d;" ("格式字符串"), w516) -> (resulting string=w515:string)  [unwired: 2 in, 1 out]
            n240 = Concatenate Strings(w515, "\r") -> (w519:string)
            n241 = call "SSI_Control.vi"("Write Buffer"=w519, "Remote Mode"=w502, "Error in (no error)"=w510, "Control"=w518, "Connection ID in"=w508) -> ("Error out"=w509:errorcluster, "Connection ID out"=w507:refnum<k5>)  [unwired: 3 in, 2 out]
            n242 = Wait (ms)(milliseconds to wait=u32 10 ("等待时间（毫秒）")) -> ()  [unwired: 1 out]
            n243 = property on="Wave" class="WFChart (严格)"("History Data"=dbl[] [] ("历史数据")) -> ()  [unwired: 2 in, 2 out]
          }
          event "Sweep": Value Change {
            n244 = event-data() -> ()  [unwired: 1 in, 5 out]
            n245 = local read "Sweep"() -> (w528:u16)
            n246 = Not Equal To 0?(x=w528) -> (x != 0?=w520:bool)
            n247 = property on="选项卡控件" class="TabCtl (严格)"("Visible"=w520) -> ()  [unwired: 2 in, 2 out]
            n248 = property on="Interval Count" class="DigNum (严格)"("Visible"=w520) -> ()  [unwired: 2 in, 2 out]
            n249 = case shown="真" w520 {
              frame False {
              }
              frame True {
                n250 = local read "Trig Mode"() -> (w530:u8)
                n251 = local read "Sweep Mode"() -> (w535:u16)
                n252 = Equal To 0?(x=w530) -> (x = 0?=w531:bool)
                n253 = Equal To 0?(x=w535) -> (x = 0?=w536:bool)
                n254 = case shown="假" w531 {
                  tunnel: [T2."Disabled and Grayed Out" ("禁用") T2."Enabled" ("禁用")] -> w533
                  tunnel: [T2."Enabled" ("禁用") T2."Disabled and Grayed Out" ("禁用")] -> w532
                  frame False {
                  }
                  frame True {
                  }
                }
                n255 = Not(x=w536) -> (.not. x?=w534:bool)
                n256 = property on="Linear Step Frequency(Hz)" class="DigNum (严格)"("Visible"=w536) -> ()  [unwired: 2 in, 2 out]
                n257 = property on="Log Step Percent(%)" class="DigNum (严格)"("Visible"=w534) -> ()  [unwired: 2 in, 2 out]
                n258 = property on="Step Time(ms)" class="DigNum (严格)"("DisabledEnum"=w533) -> ()  [unwired: 2 in, 2 out]
                n259 = property on="Interval Count" class="DigNum (严格)"("DisabledEnum"=w532) -> ()  [unwired: 2 in, 2 out]
              }
            }
            n260 = property on="Wave" class="WFChart (严格)"("History Data"=dbl[] [] ("历史数据")) -> ()  [unwired: 2 in, 2 out]
          }
        }
        n261 = local read "Connect"() -> (w37:bool)
        n262 = Not(x=w37) -> (.not. x?=w47:bool)
        n263 = Or(x=w34, y=w47) -> (x .or. y?=w46:bool)
      }
      n264 = call "SSI_Close.vi"("Error in (no error)"=w28, "Connection ID in"=w24) -> ("Error out"=→"Error out":errorcluster)  [unwired: 5 in]
    }
  }
